vi "Set Symbols Selection.vi"(7 "Indices Modified":i32[](array[numeric]), 8 "error in (no error)":errorcluster, 10 "Selected Items In":bool[](array[boolean]), 11 "Listbox or Tree":refnum<vi>) -> (0 "error out":errorcluster, 2 "Selected Items Out":bool[](array[boolean]))   [LabVIEW 2024]
doc: "This VI will change the symbols of a <B>Listbox or Tree</B> to make them appear as if items are selected based on the <B>Selected Items</B> for that control. This VI accepts a generic Control Ref but only a single column, multicolumn listbox, or tree controls will work without error.\n-------------\nBrian Hoover (hooovahh)"
uses:
  <userlib>/_OpenG.lib/array/array.llb/Remove Duplicates from 1D Array (String)__ogtk.vi
  <userlib>/_OpenG.lib/array/array.llb/Sort 1D Array (I32)__ogtk.vi
  <userlib>/_OpenG.lib/array/array.llb/Reorder 1D Array2 (String)__ogtk.vi
  <userlib>/_OpenG.lib/array/array.llb/openg_array.lvlib
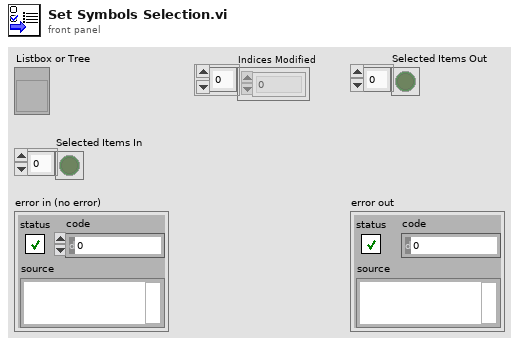
[diagram p1: front panel]
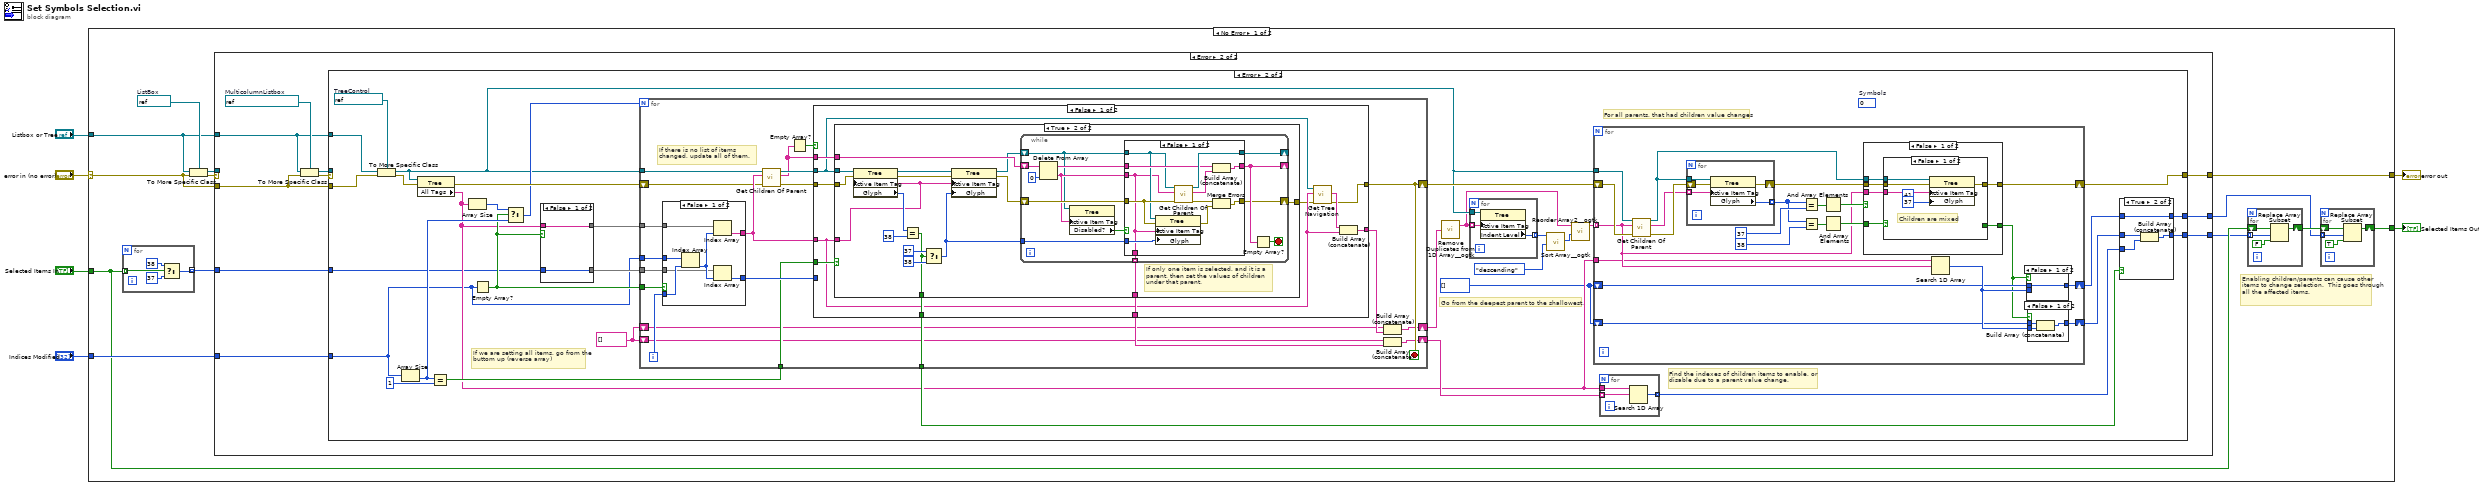
[diagram p0: block diagram]
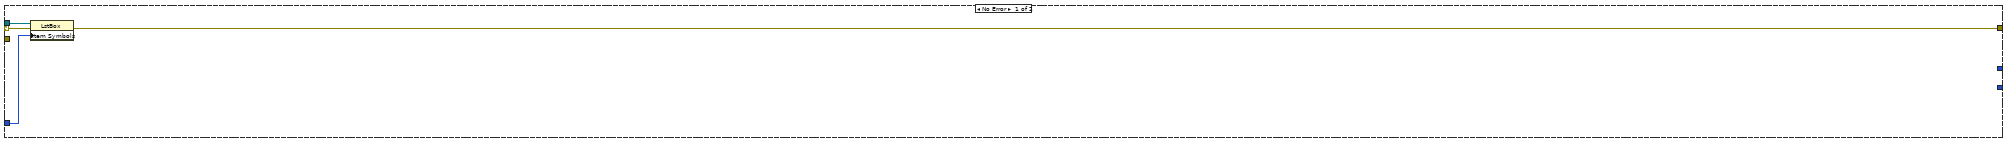
[diagram p2: hidden frame]
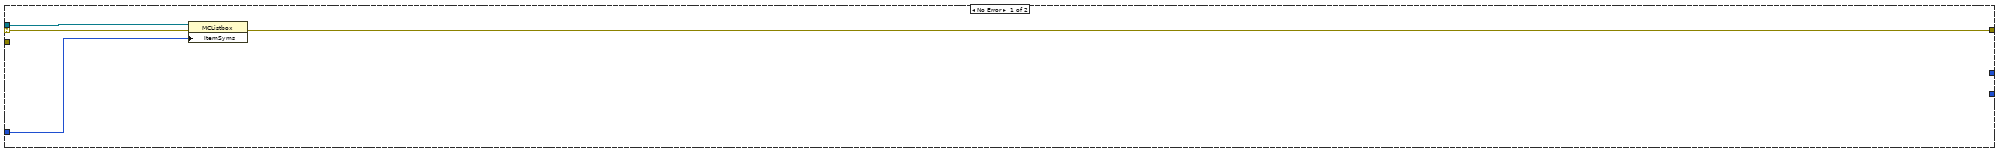
[diagram p3: hidden frame]
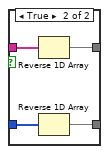
[diagram p4: hidden frame]
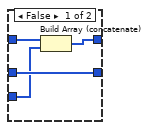
[diagram p5: hidden frame]
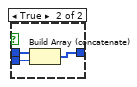
[diagram p6: hidden frame]
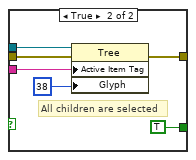
[diagram p8: hidden frame]
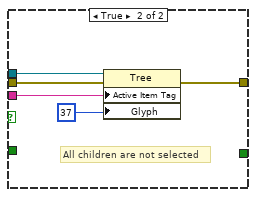
[diagram p9: hidden frame]
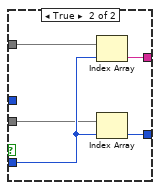
[diagram p10: hidden frame]
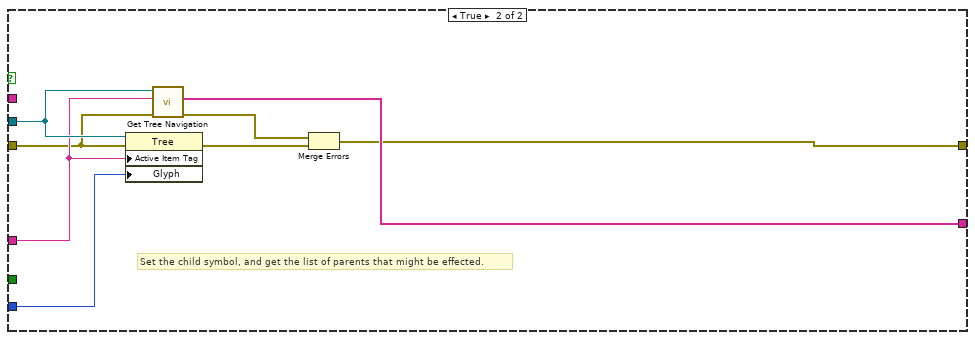
[diagram p13: hidden frame]
diagram:
  n1 = case shown="No Error" "error in (no error)" {
    selector: "error in (no error)" -> [w14 w259]
    tunnel: [w19 w259] -> w6
    tunnel: "Selected Items In" -> [w11 w258]
    tunnel: "Listbox or Tree" -> [w13 _]
    tunnel: "Indices Modified" -> [w12 _]
    tunnel: [w7 w258] -> w1
    frame No Error {
      w15 = refnum<vi> refnum  # ListBox
      # "Enabling children/parents can cause other items to change selection.  This goes through all the affected items."
      n2 = for {
        tunnel: w11 -> [w31] mode=indexing
        tunnel: [w28] -> w18 mode=indexing
        n3 = Select(t=38, s=w31, f=37) -> (s? t:f=w28:i32)
      }
      n4 = To More Specific Class(target class=w15, reference=w13, error in=w14) -> (specific class reference=w17:refnum<vi>, error out=w16:errorcluster)
      n5 = case shown="Error" w16 {
        selector: w16 -> [w34 _]
        tunnel: w17 -> [w35 _]
        tunnel: w18 -> [w33 w44]
        tunnel: w14 -> [_ w40]
        tunnel: [w32 w43] -> w19
        tunnel: w13 -> [_ w39]
        tunnel: w12 -> [_ w38]
        tunnel: [_ w37] -> w10
        tunnel: [_ w36] -> w8
        frame No Error {
          n6 = property class="LstBox"(reference=w35, error in=w34, "Item Symbols"=w33) -> (error out=w32:errorcluster)  [unwired: 1 out]
        }
        frame Error {
          w45 = refnum<vi> refnum  # MulticolumnListbox
          n7 = To More Specific Class(target class=w45, reference=w39, error in=w40) -> (specific class reference=w42:refnum<vi>, error out=w41:errorcluster)
          n8 = case shown="Error" w41 {
            selector: w41 -> [w46 _]
            tunnel: w44 -> [w49 w61]
            tunnel: [w48 w77] -> w43
            tunnel: w42 -> [w47 _]
            tunnel: w40 -> [_ w82]
            tunnel: w39 -> [_ w81]
            tunnel: w38 -> [_ w58]
            tunnel: [_ w65] -> w37
            tunnel: [_ w64] -> w36
            frame No Error {
              n9 = property class="MCListbox"(reference=w47, error in=w46, "ItemSyms"=w49) -> (error out=w48:errorcluster)  [unwired: 1 out]
            }
            frame Error {
              (unwired) 0  # Symbols
              w57 = string[] []
              w56 = i32[] [] ("Array")
              w83 = refnum<vi> refnum  # TreeControl
              # "Go from the deepest parent to the shallowest."
              # "For all parents, that had children value changes"
              # "Find the indexes of children items to enable, or disable due to a parent value change."
              # "If we are setting all items, go from the buttom up (reverse array)"
              n10 = To More Specific Class(target class=w83, reference=w81, error in=w82) -> (specific class reference=w55:refnum<vi>, error out=w80:errorcluster)
              n11 = Array Size(array=w58) -> (size(s)=w72:i32)
              n12 = property class="Tree"(reference=w55, error in=w80) -> (error out=w79:errorcluster, "All Tags"=w62:string[])  [unwired: 1 out]
              n13 = Equal?(x=w72, y=1) -> (x = y?=w74:bool)
              n14 = Array Size(array=w62) -> (size(s)=w73:i32)
              n15 = Empty Array?(array=w58) -> (empty?=w63:bool)
              n16 = Select(t=w73, s=w63, f=w72) -> (s? t:f=w71:i32)
              n17 = case shown="False" w63 {
                tunnel: w62 -> [w88 w92]
                tunnel: w61 -> [w87 w91]
                tunnel: [w88 w90] -> w60
                tunnel: [w87 w89] -> w59
                frame False {
                }
                frame True {
                  n18 = Reverse 1D Array(array=w92) -> (reversed array=w90:string[])
                  n19 = Reverse 1D Array(array=w91) -> (reversed array=w89:i32[])
                }
              }
              n20 = for {
                N: w71 -> [_]
                tunnel: w55 -> [w182]
                tunnel: w60 -> [w173]
                shift-right: [w180] -> w78
                shift-left: w79 -> [w166]
                tunnel: w74 -> [w174]
                tunnel: w58 -> [w170]
                tunnel: w63 -> [w169]
                tunnel: [w167] -> w69
                tunnel: w59 -> [w165]
                shift-right: [w163] -> w76
                shift-left: w57 -> [w164]
                shift-right: [w161] -> w70
                shift-left: w57 -> [w162]
                i -> [w168]
                stop <- w180 stop-if-true
                # "If there is no list of items changed, update all of them."
                n21 = case shown="False" w169 {
                  tunnel: [w189 w194] -> w177
                  tunnel: w173 -> [w188 w190]
                  tunnel: [w187 w193] -> w172
                  tunnel: w170 -> [w186 _]
                  tunnel: w168 -> [w184 w192]
                  tunnel: w165 -> [w183 w191]
                  frame False {
                    n22 = Index Array(array=w186, index=w184) -> (element=w185:i32)
                    n23 = Index Array(array=w188, index=w185) -> (element=w187:string)
                    n24 = Index Array(array=w183, index=w185) -> (element=w189:i32)
                  }
                  frame True {
                    n25 = Index Array(array=w190, index=w192) -> (element=w193:string)
                    n26 = Index Array(array=w191, index=w192) -> (element=w194:i32)
                  }
                }
                n27 = call "Get Children Of Parent.vi"("error in (no error)"=w166, "Parent Tag"=w172, "Tree Ref In"=w182) -> ("error out"=w179:errorcluster, "Children Tags"=w176:string[], "Tree Ref Out"=w178:refnum<vi>)  [unwired: 5 in, 1 out]
                n28 = Empty Array?(array=w176) -> (empty?=w181:bool)
                n29 = case shown="False" w181 {
                  tunnel: [w195 w251] -> w180
                  tunnel: w179 -> [w202 w252]
                  tunnel: w178 -> [w198 w255]
                  tunnel: w177 -> [_ w257]
                  tunnel: w172 -> [w199 w254]
                  tunnel: w176 -> [w201 _]
                  tunnel: [w204 w253] -> w175
                  tunnel: w174 -> [w203 _]
                  tunnel: [w205 _] -> w171
                  tunnel: [w200 _] -> w167
                  frame False {
                    n30 = case shown="True" w203 {
                      tunnel: w202 -> [w206 w215]
                      tunnel: [w206 w222] -> w196
                      tunnel: [_ w221] -> w205
                      tunnel: w198 -> [_ w216]
                      tunnel: w199 -> [_ w207]
                      tunnel: w201 -> [_ w214]
                      tunnel: [_ w213] -> w200
                      frame False {
                        # "A parent was changed, but multiple things were changed, so no need to update the children."
                      }
                      frame True {
                        # "If only one item is selected, and it is a parent, then set the values of children under that parent."
                        n31 = property class="Tree"(reference=w216, error in=w215, "Active Item Tag"=w207) -> (reference out=w210:refnum<vi>, error out=w211:errorcluster, "Glyph"=w219:i32)
                        n32 = Equal?(x=w219, y=38) -> (x = y?=w213:bool)
                        n33 = Select(t=37, s=w213, f=38) -> (s? t:f=w208:i32)
                        n34 = property class="Tree"(reference=w210, error in=w211, "Active Item Tag"=w207, "Glyph"=w208) -> (reference out=w209:refnum<vi>, error out=w212:errorcluster)
                        n35 = while {
                          shift-right: [w230] -> _
                          shift-left: w214 -> [w235]
                          shift-right: [w227] -> w222
                          shift-left: w212 -> [w231]
                          shift-right: [w233] -> _
                          shift-left: w209 -> [w225]
                          tunnel: [w223] -> w221 mode=indexing
                          tunnel: w208 -> [w228]
                          stop <- w229 stop-if-true
                          n36 = Delete From Array(array=w235, index=0) -> (deleted portion=w226:string, array with subset deleted=w232:string[])  [unwired: 1 in]
                          n37 = property class="Tree"(reference=w225, "Active Item Tag"=w226) -> ("Disabled?"=w224:bool)  [unwired: 1 in, 2 out]
                          n38 = case shown="False" w224 {
                            tunnel: [w246 w249] -> w233
                            tunnel: w232 -> [w245 w248]
                            tunnel: w231 -> [w242 w247]
                            tunnel: [w241 w248] -> w230
                            tunnel: w228 -> [w240 _]
                            tunnel: [w239 w247] -> w227
                            tunnel: w226 -> [w236 _]
                            tunnel: w225 -> [w237 w249]
                            tunnel: [w236 _] -> w223
                            frame False {
                              n39 = property class="Tree"(reference=w237, error in=w242, "Active Item Tag"=w236, "Glyph"=w240) -> (error out=w238:errorcluster)  [unwired: 1 out]
                              n40 = call "Get Children Of Parent.vi"("error in (no error)"=w242, "Parent Tag"=w236, "Tree Ref In"=w237) -> ("error out"=w243:errorcluster, "Children Tags"=w244:string[], "Tree Ref Out"=w246:refnum<vi>)  [unwired: 5 in, 1 out]
                              n41 = Build Array (concatenate)(w245, w244) -> (w241:string[])
                              n42 = Merge Errors(w243, w238) -> (w239:errorcluster)
                            }
                            frame True {
                            }
                          }
                          n43 = Empty Array?(array=w230) -> (empty?=w229:bool)
                        }
                      }
                    }
                    n44 = call "Get Tree Navigation.vi"("error in (no error)"=w196, "Tag"=w199, "Tree Ref In"=w198) -> ("error out"=w195:errorcluster, "Parent Tags"=w197:string[])  [unwired: 5 in, 2 out]
                    n45 = Build Array (concatenate)(w197, w199) -> (w204:string[])
                  }
                  frame True {
                    # "Set the child symbol, and get the list of parents that might be effected."
                    n46 = property class="Tree"(reference=w255, error in=w252, "Active Item Tag"=w254, "Glyph"=w257) -> (error out=w256:errorcluster)  [unwired: 1 out]
                    n47 = call "Get Tree Navigation.vi"("error in (no error)"=w252, "Tag"=w254, "Tree Ref In"=w255) -> ("error out"=w250:errorcluster, "Parent Tags"=w253:string[])  [unwired: 5 in, 2 out]
                    n48 = Merge Errors(w250, w256) -> (w251:errorcluster)
                  }
                }
                n49 = Build Array (concatenate)(w164, w175) -> (w163:string[])
                n50 = Build Array (concatenate)(w162, w171) -> (w161:string[])
              }
              n51 = call-poly <userlib>:"Remove Duplicates from 1D Array__ogtk.vi"("Input Array"=w76) -> ("Output Array"=w52:string[])  [unwired: 1 out]
              n52 = for {
                tunnel: w52 -> [w86] mode=indexing
                tunnel: [w85] -> w54 mode=indexing
                tunnel: w55 -> [w84]
                n53 = property class="Tree"(reference=w84, "Active Item Tag"=w86) -> ("Indent Level"=w85:i32)  [unwired: 1 in, 2 out]
              }
              n54 = call-poly <userlib>:"Sort Array__ogtk.vi"("Order"=enum16{"ascending", "descending"}."descending", "Array in"=w54) -> ("Sorted Pointers"=w51:i32[])  [unwired: 8 in, 1 out]
              n55 = call-poly <userlib>:"Reorder Array2__ogtk.vi"("indices"=w51, "array"=w52) -> ("reordered array"=w50:string[])  [unwired: 9 in]
              n56 = for {
                tunnel: w55 -> [w123]
                tunnel: w50 -> [w111] mode=indexing
                shift-right: [w120] -> w77
                shift-left: w78 -> [w125]
                tunnel: w62 -> [w110]
                shift-right: [w107] -> w67
                shift-left: w56 -> [w108]
                shift-right: [w105] -> w66
                shift-left: w56 -> [w106]
                n57 = call "Get Children Of Parent.vi"("error in (no error)"=w125, "Parent Tag"=w111, "Tree Ref In"=w123) -> ("error out"=w124:errorcluster, "Children Tags"=w122:string[], "Tree Ref Out"=w118:refnum<vi>)  [unwired: 5 in, 1 out]
                n58 = for {
                  tunnel: w118 -> [w159]
                  tunnel: w122 -> [w157] mode=indexing
                  shift-right: [w160] -> w119
                  shift-left: w124 -> [w158]
                  tunnel: [w156] -> w114 mode=indexing
                  n59 = property class="Tree"(reference=w159, error in=w158, "Active Item Tag"=w157) -> (error out=w160:errorcluster, "Glyph"=w156:i32)  [unwired: 1 out]
                }
                n60 = Equal?(x=w114, y=37) -> (x = y?=w115:bool[])
                n61 = Equal?(x=w114, y=38) -> (x = y?=w116:bool[])
                n62 = And Array Elements(Boolean array=w115) -> (logical AND=w117:bool)
                n63 = And Array Elements(Boolean array=w116) -> (logical AND=w112:bool)
                n64 = case shown="False" w117 {
                  tunnel: [w136 w155] -> w120
                  tunnel: w119 -> [w139 w154]
                  tunnel: w118 -> [w138 w153]
                  tunnel: w111 -> [w137 w152]
                  tunnel: w112 -> [w135 _]
                  tunnel: [w134 _] -> w104
                  frame False {
                    n65 = case shown="False" w135 {
                      tunnel: w139 -> [w142 w149]
                      tunnel: w138 -> [w143 w148]
                      tunnel: w137 -> [w140 w147]
                      tunnel: [w141 w146] -> w136
                      tunnel: [_ TRUE] -> w134
                      frame False {
                        (unwired) 41
                        # "Children are mixed"
                        n66 = property class="Tree"(reference=w143, error in=w142, "Active Item Tag"=w140, "Glyph"=37) -> (error out=w141:errorcluster)  [unwired: 1 out]
                      }
                      frame True {
                        # "All children are selected"
                        n67 = property class="Tree"(reference=w148, error in=w149, "Active Item Tag"=w147, "Glyph"=38) -> (error out=w146:errorcluster)  [unwired: 1 out]
                      }
                    }
                  }
                  frame True {
                    # "All children are not selected"
                    n68 = property class="Tree"(reference=w153, error in=w154, "Active Item Tag"=w152, "Glyph"=37) -> (error out=w155:errorcluster)  [unwired: 1 out]
                  }
                }
                n69 = Search 1D Array(1D array=w110, element=w111) -> (index of element=w109:i32)  [unwired: 1 in]
                n70 = case shown="False" w104 {
                  tunnel: w106 -> [w126 w128]
                  tunnel: w109 -> [_ w127]
                  tunnel: [w126 w129] -> w105
                  frame False {
                  }
                  frame True {
                    n71 = Build Array (concatenate)(w128, w127) -> (w129:i32[])
                  }
                }
                n72 = case shown="False" w104 {
                  tunnel: w108 -> [w131 w133]
                  tunnel: w109 -> [w130 _]
                  tunnel: [w132 w133] -> w107
                  frame False {
                    n73 = Build Array (concatenate)(w131, w130) -> (w132:i32[])
                  }
                  frame True {
                  }
                }
              }
              n74 = for {
                tunnel: w70 -> [w103] mode=indexing
                tunnel: w62 -> [w102]
                tunnel: [w101] -> w68 mode=indexing
                n75 = Search 1D Array(1D array=w102, element=w103) -> (index of element=w101:i32)  [unwired: 1 in]
              }
              n76 = case shown="True" w69 {
                tunnel: w68 -> [w93 w99]
                tunnel: w67 -> [w94 w100]
                tunnel: [w94 w98] -> w65
                tunnel: [w95 w97] -> w64
                tunnel: w66 -> [w96 w97]
                frame False {
                  n77 = Build Array (concatenate)(w96, w93) -> (w95:i32[])
                }
                frame True {
                  n78 = Build Array (concatenate)(w100, w99) -> (w98:i32[])
                }
              }
            }
          }
        }
      }
      n79 = for {
        shift-right: [w26] -> w9
        shift-left: w11 -> [w27]
        tunnel: w10 -> [w24] mode=indexing
        n80 = Replace Array Subset(array=w27, new element=FALSE ("new element/subarray"), index=w24) -> (w26:bool[])
      }
      n81 = for {
        shift-right: [w22] -> w7
        shift-left: w9 -> [w23]
        tunnel: w8 -> [w20] mode=indexing
        n82 = Replace Array Subset(array=w23, new element=TRUE ("new element/subarray"), index=w20) -> (w22:bool[])
      }
    }
    frame Error {
    }
  }
  "error out" <- w6
  "Selected Items Out" <- w1
